vi "Station2_Data_Log_Bypass_Station1.vi"(8 "error in (no error)":errorcluster, 11 "Cluster 2":T2) -> (0 "error out":errorcluster)   [LabVIEW 2017]
uses:
  <vilib>/addons/database/Connection.llb/Conn ObjectReference.ctl
  <vilib>/addons/database/NI_Database_API.lvlib
panel:
  # "bypass station1 ..."
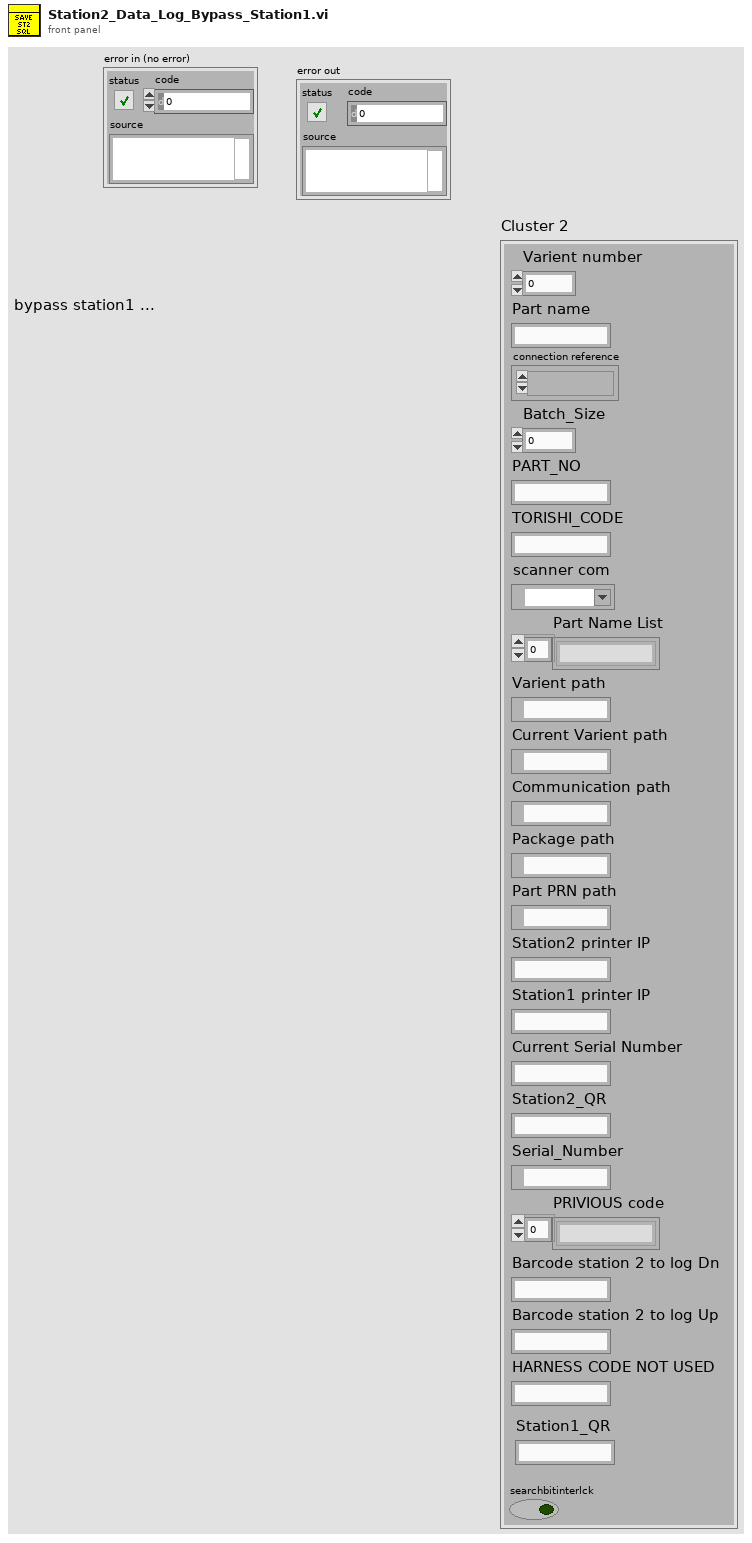
[diagram p1: front panel]
types:
  T1 = typedef "NI_Database_API.lvlib/Conn ObjectReference.ctl" = refnum<k1>
  T2 = cluster{"Varient number":u16, "Part name":string, "connection reference":T1, "Batch_Size":u16, "PART_NO":string, "TORISHI_CODE":string, "scanner com":refnum<visa-resource-name>, "Part Name List":string[], "Varient path":path, "Current Varient path":path, "Communication path":path, "Package path":path, "Part PRN path":path, "Station2 printer IP":string, "Station1 printer IP":string, "Current Serial Number":string, "Station2_QR":string, "Serial_Number":path, "PRIVIOUS code":string[], "Barcode station 2 to log Dn":string, "Barcode station 2 to log Up":string, "HARNESS CODE NOT USED":string, "Station1_QR":string, "searchbitinterlck":bool}
  T3 = cluster{"appended array[0]":string, "appended array[1]":string, "appended array[2]":string, "appended array[3]":string, "appended array[4]":string, "appended array[5]":string, "appended array[6]":string, "appended array[7]":string, "appended array[8]":string, "appended array[9]":string, "appended array[10]":string, "appended array[11]":string, "appended array[12]":string, "appended array[13]":string, "appended array[14]":string, "appended array[15]":string, "appended array[16]":string, "appended array[17]":string, "appended array[18]":string, "appended array[19]":string, "appended array[20]":string, "appended array[21]":string, "appended array[22]":string, "appended array[23]":string, "appended array[24]":string, "appended array[25]":string, "appended array[26]":string, "appended array[27]":string, "appended array[28]":string, "appended array[29]":string, "appended array[30]":string, "appended array[31]":string, "appended array[32]":string, "appended array[33]":string, "appended array[34]":string, "appended array[35]":string, "appended array[36]":string, "appended array[37]":string, "appended array[38]":string, "appended array[39]":string, "appended array[40]":string, "appended array[41]":string, "appended array[42]":string, "appended array[43]":string, "appended array[44]":string, "appended array[45]":string, "appended array[46]":string, "appended array[47]":string, "appended array[48]":string, "appended array[49]":string, "appended array[50]":string, "appended array[51]":string, "appended array[52]":string, "appended array[53]":string, "appended array[54]":string, "appended array[55]":string, "appended array[56]":string, "appended array[57]":string, "appended array[58]":string, "appended array[59]":string, "appended array[60]":string, "appended array[61]":string, "appended array[62]":string, "appended array[63]":string, "appended array[64]":string, "appended array[65]":string, "appended array[66]":string, "appended array[67]":string, "appended array[68]":string, "appended array[69]":string, "appended array[70]":string, "appended array[71]":string, "appended array[72]":string, "appended array[73]":string, "appended array[74]":string, "appended array[75]":string, "appended array[76]":string}
  T4 = typedef "LVDateTimeRec.ctl" = cluster{"fractional second":dbl, "second":i32, "minute":i32, "hour":i32, "day of month":i32, "month":i32, "year":i32, "day of week":i32, "day of year":i32, "DST":i32}
  T5 = cluster{"time stamp":timestamp, string, string, string, string, string, string, string, string, string, string, string, string, string, string, string, string, string, string, string, string, string, string, string, string, string, string, string, string, string, string, string, string, "time stamp":timestamp, "Station2_QR":string, string, string, "Numeric 2":string, "Numeric 2":string, "Numeric 2":string, string, "Numeric 2":string, "Numeric 2":string, string, "Numeric 2":string, "Numeric 2":string, "Numeric 2":string, string, "Numeric 2":string, "Numeric 2":string, "Numeric 2":string, string, "Numeric 2":string, "Numeric 2":string, "Numeric 2":string, string, "Numeric 2":string, "Numeric 2":string, "Numeric 2":string, string, "Numeric 2":string, "Numeric 2":string, "Numeric 2":string, string, "Numeric 2":string, "Numeric 2":string, "Numeric 2":string, string, string, string, string, string, string, string, string, string, string}
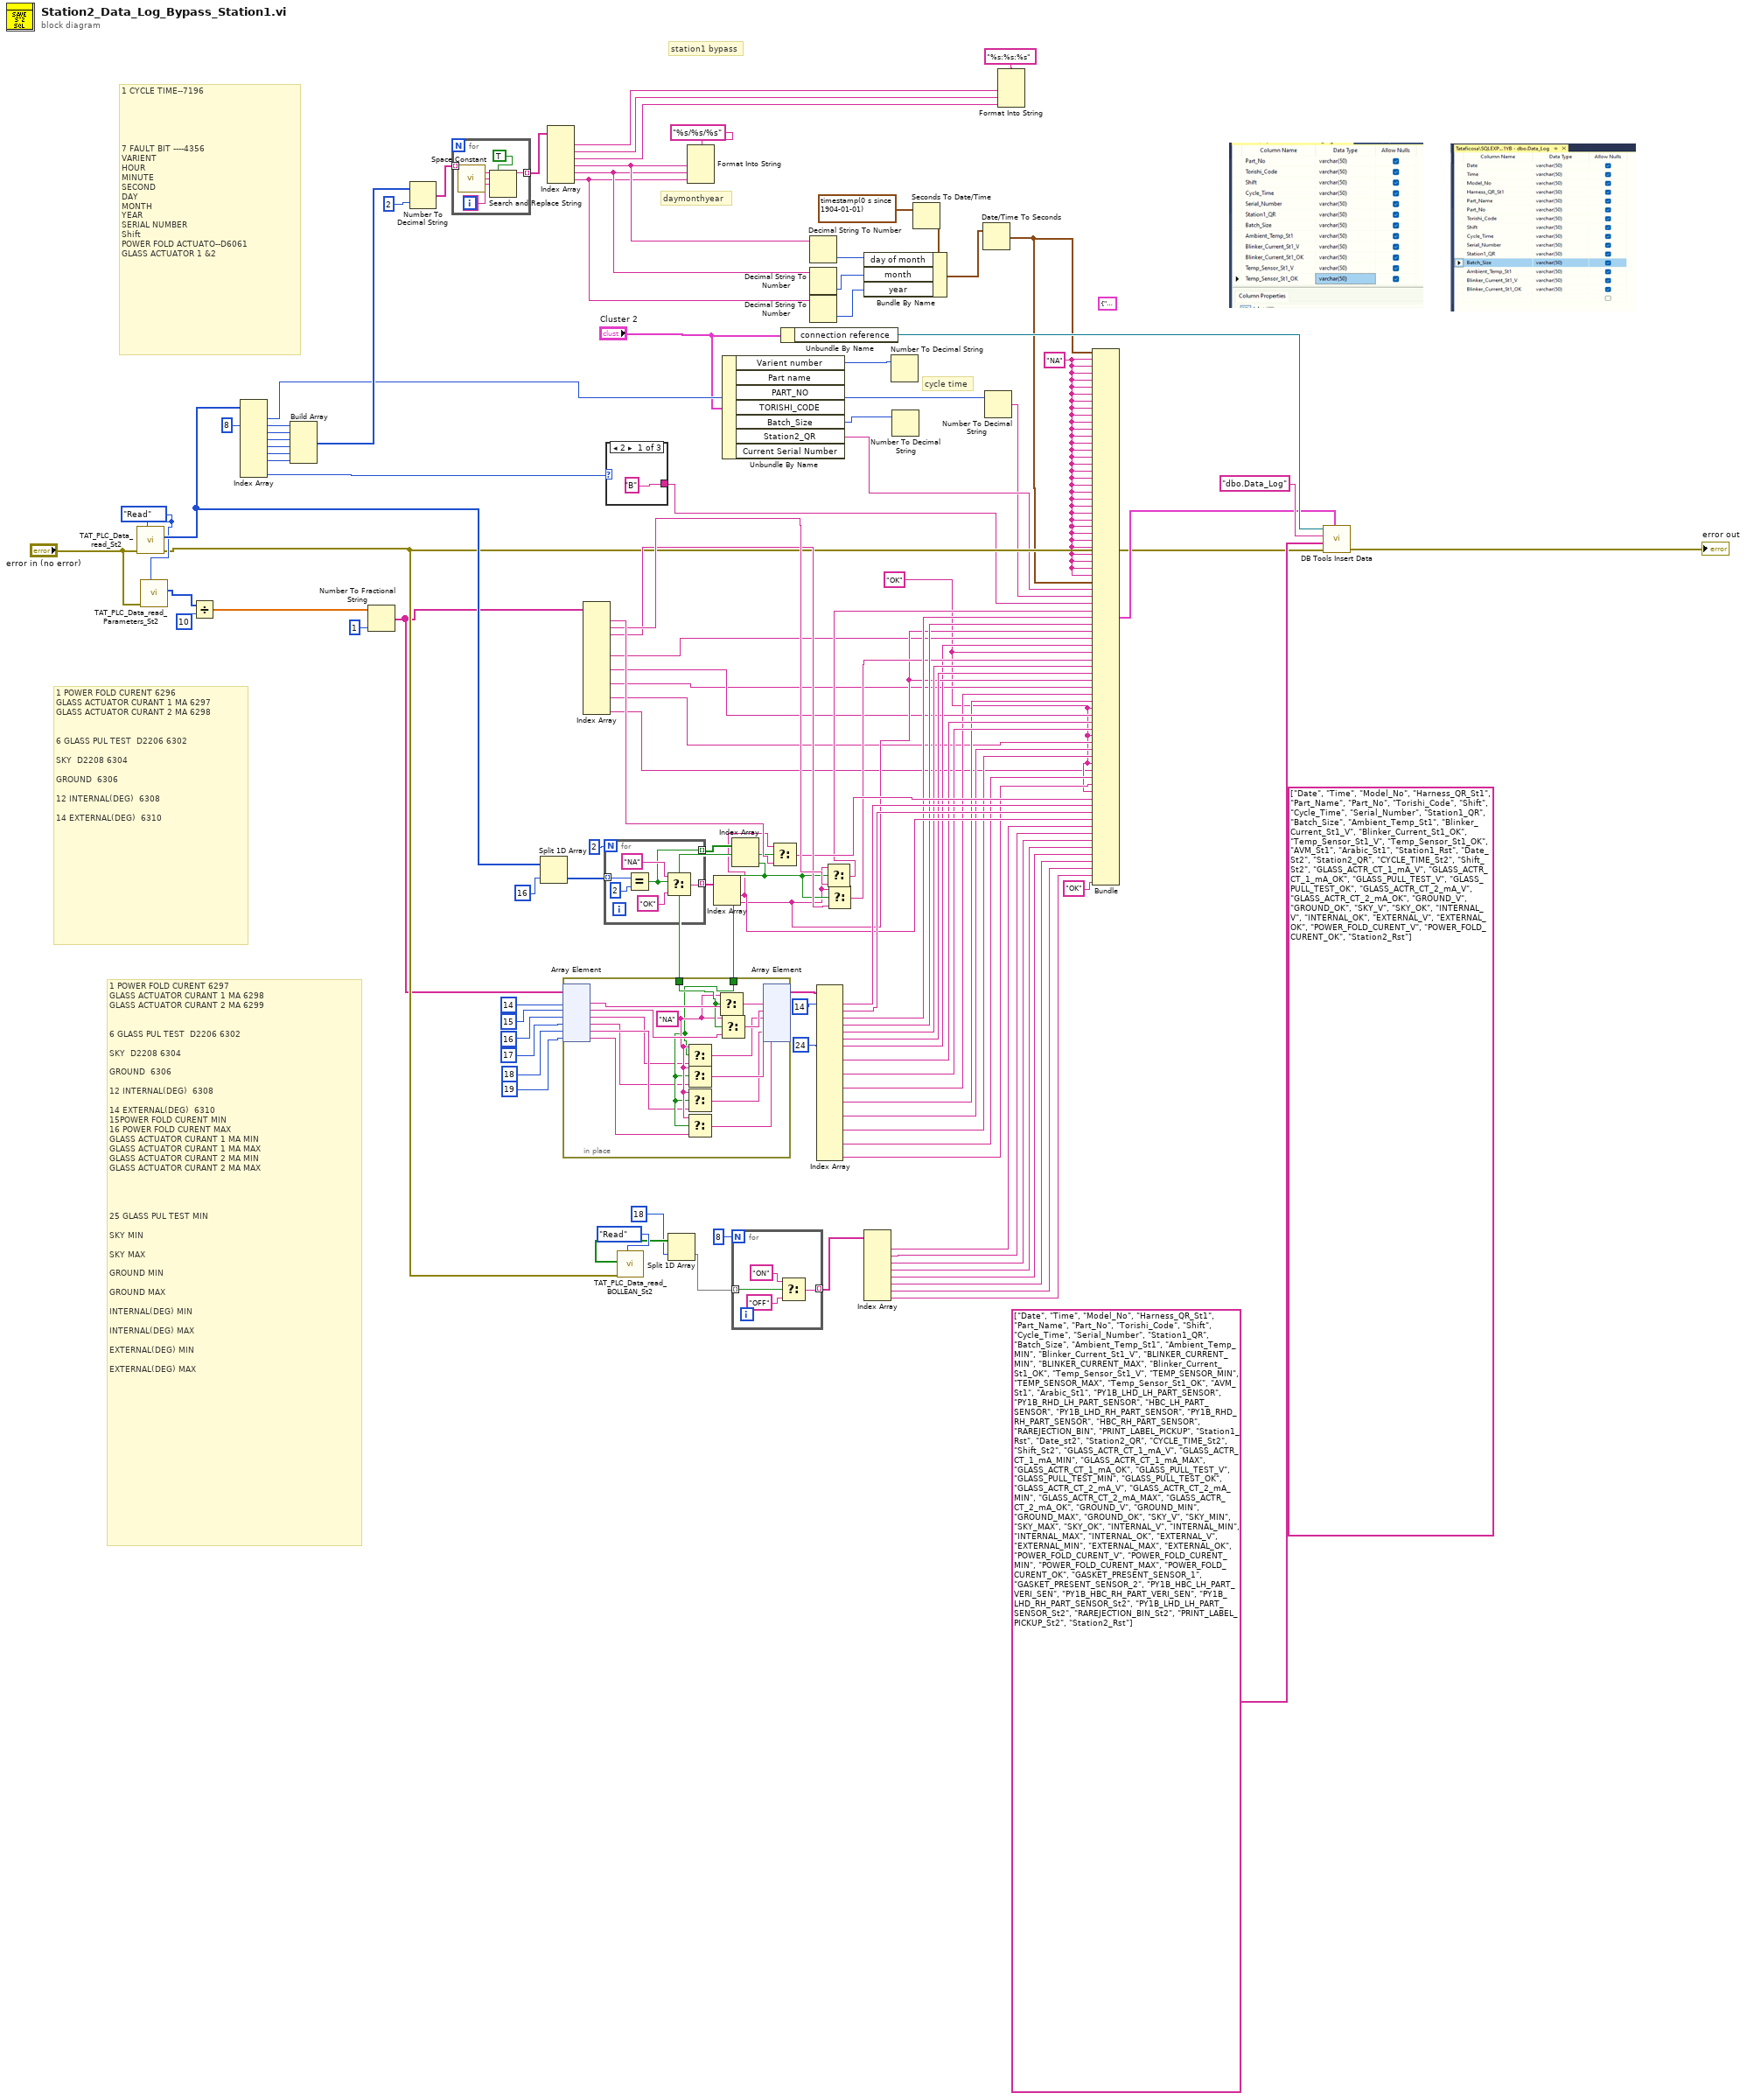
[diagram p0: block diagram]
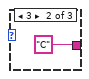
[diagram p2: hidden frame]
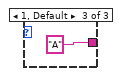
[diagram p3: hidden frame]
diagram:
  (unwired) T3 {"appended array[0]"="Date", "appended array[1]"="Time", "appended array[2]"="Model_No", "appended array[3]"="Harness_QR_St1", "appended array[4]"="Part_Name", "appended array[5]"="Part_No", "appended array[6]"="Torishi_Code", "appended array[7]"="Shift", "appended array[8]"="Cycle_Time", "appended array[9]"="Serial_Number", "appended array[10]"="Station1_QR", "appended array[11]"="Batch_Size", "appended array[12]"="Ambient_Temp_St1", "appended array[13]"="Ambient_Temp_MIN", "appended array[14]"="Blinker_Current_St1_V", "appended array[15]"="BLINKER_CURRENT_MIN", "appended array[16]"="BLINKER_CURRENT_MAX", "appended array[17]"="Blinker_Current_St1_OK", "appended array[18]"="Temp_Sensor_St1_V", "appended array[19]"="TEMP_SENSOR_MIN", "appended array[20]"="TEMP_SENSOR_MAX", "appended array[21]"="Temp_Sensor_St1_OK", "appended array[22]"="AVM_St1", "appended array[23]"="Arabic_St1", "appended array[24]"="PY1B_LHD_LH_PART_SENSOR", "appended array[25]"="PY1B_RHD_LH_PART_SENSOR", "appended array[26]"="HBC_LH_PART_SENSOR", "appended array[27]"="PY1B_LHD_RH_PART_SENSOR", "appended array[28]"="PY1B_RHD_RH_PART_SENSOR", "appended array[29]"="HBC_RH_PART_SENSOR", "appended array[30]"="RAREJECTION_BIN", "appended array[31]"="PRINT_LABEL_PICKUP", "appended array[32]"="Station1_Rst", "appended array[33]"="Date_st2", "appended array[34]"="Station2_QR", "appended array[35]"="CYCLE_TIME_St2", "appended array[36]"="Shift_St2", "appended array[37]"="GLASS_ACTR_CT_1_mA_V", "appended array[38]"="GLASS_ACTR_CT_1_mA_MIN", "appended array[39]"="GLASS_ACTR_CT_1_mA_MAX", "appended array[40]"="GLASS_ACTR_CT_1_mA_OK", "appended array[41]"="GLASS_PULL_TEST_V", "appended array[42]"="GLASS PUL TEST_MIN", "appended array[43]"="GLASS_PULL_TEST_OK", "appended array[44]"="GLASS_ACTR_CT_2_mA_V", "appended array[45]"="GLASS_ACTR_CT_2_mA_MIN", "appended array[46]"="GLASS_ACTR_CT_2_mA_MAX", "appended array[47]"="GLASS_ACTR_CT_2_mA_OK", "appended array[48]"="GROUND_V", "appended array[49]"="GROUND_MIN", "appended array[50]"="GROUND_MAX", "appended array[51]"="GROUND_OK", "appended array[52]"="SKY_V", "appended array[53]"="SKY_MIN", "appended array[54]"="SKY_MAX", "appended array[55]"="SKY_OK", "appended array[56]"="INTERNAL_V", "appended array[57]"="INTERNAL_MIN", "appended array[58]"="INTERNAL_MAX", "appended array[59]"="INTERNAL_OK", "appended array[60]"="EXTERNAL_V", "appended array[61]"="EXTERNAL_MIN", "appended array[62]"="EXTERNAL_MAX", "appended array[63]"="EXTERNAL_OK", "appended array[64]"="POWER_FOLD_CURENT_V", "appended array[65]"="POWER_FOLD_CURENT_MIN", "appended array[66]"="POWER_FOLD_CURENT_MAX", "appended array[67]"="POWER_FOLD_CURENT_OK", "appended array[68]"="GASKET_PRESENT_SENSOR_1", "appended array[69]"="GASKET_PRESENT_SENSOR_2", "appended array[70]"="PY1B_&_HBC_LH_PART_VERIFICATION_SENSOR_St2", "appended array[71]"="PY1B_&_HBC_RH_PART_VERIFICATION_SENSOR_St2", "appended array[72]"="PY1B_LHD_RH_PART_SENSOR_St2", "appended array[73]"="PY1B_LHD_LH_PART_SENSOR_St2", "appended array[74]"="RAREJECTION_BIN_St2", "appended array[75]"="PRINT_LABEL_PICKUP_St2", "appended array[76]"="Station2_Rst"} ("cluster")
  w2 = "NA"
  w16 = "OK"
  w78 = enum16{"Read", "Write"}."Read" ("Enum")
  (unwired) string[] ["Date", "Time", "Model_No", "Harness_QR_St1", "Part_Name", "Part_No", "Torishi_Code", "Shift", "Cycle_Time", "Serial_Number", "Station1_QR", "Batch_Size", "Ambient_Temp_St1", "Blinker_Current_St1_V", "Blinker_Current_St1_OK", "Temp_Sensor_St1_V", "Temp_Sensor_St1_OK", "AVM_St1", "Arabic_St1", "Station1_Rst", "Date_St2", "Station2_QR", "CYCLE_TIME_St2", "Shift_St2", "GLASS_ACTR_CT_1_mA_V", "GLASS_ACTR_CT_1_mA_OK", "GLASS_PULL_TEST_V", "GLASS_PULL_TEST_OK", "GLASS_ACTR_CT_2_mA_V", "GLASS_ACTR_CT_2_mA_OK", "GROUND_V", "GROUND_OK", "SKY_V", "SKY_OK", "INTERNAL_V", "INTERNAL_OK", "EXTERNAL_V", "EXTERNAL_OK", "POWER_FOLD_CURENT_V", "POWER_FOLD_CURENT_OK", "Station2_Rst"] ("columns")
  # "1 POWER FOLD CURENT 6297\nGLASS ACTUATOR CURANT 1 MA 6298\nGLASS ACTUATOR CURANT 2 MA 6299\n\n\n6 GLASS PUL TEST  D2206 6302\n\nSKY  D2208 6304\n\nGROUND  6306\n\n12 INTERNAL(DEG)  6308\n\n14 EXTERNAL(DEG)  6310\n15POWER FOLD CURENT MIN\n16 POWER FOLD CURENT MAX\nGLASS ACTUATOR CURANT 1 MA MIN\nGLASS ACTUATOR CURANT 1 MA MAX\nGLASS ACTUATOR CURANT 2 MA MIN\nGLASS ACTUATOR CURANT 2 MA MAX\n\n\n\n\n25 GLASS PUL TEST MIN\n\nSKY MIN\n\nSKY MAX\n\nGROUND MIN\n\nGROUND MAX\n\nINTERNAL(DEG) MIN\n\nINTERNAL(DEG) MAX\n\nEXTERNAL(DEG) MIN\n\nEXTERNAL(DEG) MAX"
  # "1 POWER FOLD CURENT 6296\nGLASS ACTUATOR CURANT 1 MA 6297\nGLASS ACTUATOR CURANT 2 MA 6298\n\n\n6 GLASS PUL TEST  D2206 6302\n\nSKY  D2208 6304\n\nGROUND  6306\n\n12 INTERNAL(DEG)  6308\n\n14 EXTERNAL(DEG)  6310"
  # "1 CYCLE TIME--7196\n\n\n\n\n\n7 FAULT BIT ----4356\nVARIENT\nHOUR\nMINUTE\nSECOND\nDAY\nMONTH\nYEAR\nSERIAL NUMBER\nShift\nPOWER FOLD ACTUATO--D6061\nGLASS ACTUATOR 1 &2"
  # "station1 bypass"
  # "daymonthyear"
  # "cycle time"
  n1 = call "TAT_PLC_Data_read_St2.vi"("Enum"=w78, "error in (no error)"="error in (no error)") -> ("error out"=w61:errorcluster, "Array 2"=w79:u16[])  [unwired: 8 in]
  n2 = call "TAT_PLC_Data_read_Parameters_St2.vi"("Enum"=w78, "error in (no error)"="error in (no error)") -> ("Array 2"=w76:u16[])  [unwired: 8 in, 1 out]
  n3 = Divide(x=w76, y=10 ("Numeric 2")) -> (x/y=w73:dbl[])
  n4 = Index Array(array=w79, index #2=8 ("index")) -> (element #1=w81:u16, element #2=w99:u16, element #3=w98:u16, element #4=w97:u16, element #5=w96:u16, element #6=w95:u16, element #7=w94:u16, element #9=w87:u16)  [unwired: 8 in, 1 out]
  n5 = Build Array(w99, w98, w97, w96, w95, w94) -> (w93:u16[])
  n6 = Number To Fractional String(number=w73, precision (6)=i16 1) -> (F-format string=w43:string[])  [unwired: 2 in]
  n7 = Number To Decimal String(number=w93, width (-)=i16 2) -> (decimal integer string=w102:string[])
  n8 = for {
    tunnel: w102 -> [w111] mode=indexing
    tunnel: [w110] -> w101 mode=indexing
    n9 = call <vilib>:"Space Constant.vi"() -> ("String"=w112:string)
    n10 = Search and Replace String(replace all?=TRUE ("replace all? (F)"), input string=w111, search string=w112, replace string="0" ("replace string (\"\")")) -> (result string=w110:string)  [unwired: 4 in, 3 out]
  }
  n11 = Split 1D Array(array=w79, index=16) -> (second subarray=w85:u16[])  [unwired: 1 out]
  n12 = Index Array(array=w101) -> (element #1=w91:string, element #2=w90:string, element #3=w89:string, element #4=w5:string, element #5=w4:string, element #6=w3:string)  [unwired: 6 in]
  n13 = Index Array(array=w43) -> (element #1=w72:string, element #2=w71:string, element #3=w70:string, element #6=w28:string, element #8=w25:string, element #10=w24:string, element #12=w21:string, element #14=w15:string)  [unwired: 14 in, 6 out]
  n14 = for {
    N: 2 -> [_]
    tunnel: w85 -> [w120] mode=indexing
    tunnel: [w116] -> w83 mode=indexing
    tunnel: [w115] -> w82 mode=indexing
    n15 = Equal?(x=w120, y=2) -> (x = y?=w115:bool)
    n16 = Select(t="NA", s=w115, f="OK") -> (s? t:f=w116:string)
  }
  n17 = case shown="2" w87 {
    tunnel: ["B" "C" "A"] -> w12
    frame 2 {
    }
    frame 3 {
    }
    frame 1, Default {
    }
  }
  n18 = call "TAT_PLC_Data_read_BOLLEAN_St2.vi"("Enum"=enum16{"Read", "Write"}."Read", "error in (no error)"=w61) -> ("Array 2"=w66:bool[])  [unwired: 8 in, 1 out]
  n19 = Split 1D Array(array=w66, index=18) -> (second subarray=w64:bool[])  [unwired: 1 out]
  n20 = Format Into String(format string="%s/%s/%s" ("time format string (%c)"), w5, w4, w3) -> ()  [unwired: 2 in, 2 out]
  n21 = Index Array(array=w83) -> (element #1=w38:string, element #2=w30:string)  [unwired: 2 in]
  n22 = Unbundle By Name("Cluster 2") -> ("Varient number"=w108:u16, "Batch_Size"=w109:u16, "Station2_QR"=w14:string)  [unwired: 4 out]
  n23 = Index Array(array=w82) -> (element #1=w42:bool, element #2=w41:bool)  [unwired: 2 in]
  n24 = in-place {
    in-place-border: w41 -> [w132]
    in-place-border: w42 -> [w134]
    w133 = "NA"
    n25 = in-place-array #1(w43, 14 ("index"), 15 ("index"), 16 ("index"), 17 ("index"), 18 ("index"), 19 ("index")) -> (w138:string, w135:string, w128:string, w129:string, w130:string, w131:string)
    n26 = Select(t=w133, s=w132, f=w128) -> (s? t:f=w127:string)
    n27 = Select(t=w133, s=w132, f=w129) -> (s? t:f=w126:string)
    n28 = Select(t=w133, s=w132, f=w130) -> (s? t:f=w125:string)
    n29 = Select(t=w133, s=w132, f=w131) -> (s? t:f=w124:string)
    n30 = Select(t=w133, s=w134, f=w138) -> (s? t:f=w137:string)
    n31 = Select(t=w133, s=w134, f=w135) -> (s? t:f=w136:string)
    n32 = in-place-array #1(w137, w136, w127, w126, w125, w124) -> (w45:string[])  [unwired: 6 out]
  }
  n33 = for {
    N: 8 -> [_]
    tunnel: w64 -> [w140] mode=indexing
    tunnel: [w139] -> w62 mode=indexing
    n34 = Select(t="ON", s=w140, f="OFF") -> (s? t:f=w139:string)
  }
  n35 = Select(t=w38, s=w42, f=w72) -> (s? t:f=w37:string)
  n36 = Unbundle By Name("Cluster 2") -> ("connection reference"=w107:T1)
  n37 = Decimal String To Number(string=w5) -> (number=w9:i32)  [unwired: 2 in, 1 out]
  n38 = Decimal String To Number(string=w4) -> (number=w8:i32)  [unwired: 2 in, 1 out]
  n39 = Decimal String To Number(string=w3) -> (number=w7:i32)  [unwired: 2 in, 1 out]
  n40 = Index Array(array=w45, index #1=14 ("index"), index #7=24 ("index")) -> (element #1=w40:string, element #2=w39:string, element #3=w36:string, element #4=w35:string, element #5=w33:string, element #6=w32:string, element #7=w29:string, element #9=w27:string, element #11=w26:string, element #13=w23:string, element #15=w22:string, element #17=w20:string, element #19=w19:string, element #21=w18:string, element #23=w17:string)  [unwired: 21 in, 8 out]
  n41 = Select(t=w30, s=w41, f=w71) -> (s? t:f=w34:string)
  n42 = Select(t=w30, s=w41, f=w70) -> (s? t:f=w31:string)
  n43 = Index Array(array=w62) -> (element #1=w53:string, element #2=w54:string, element #3=w55:string, element #4=w56:string, element #5=w57:string, element #6=w58:string, element #7=w59:string, element #8=w60:string)  [unwired: 8 in]
  n44 = Number To Decimal String(number=w108) -> ()  [unwired: 1 in, 1 out]
  n45 = Number To Decimal String(number=w109) -> ()  [unwired: 1 in, 1 out]
  n46 = Seconds To Date/Time(time stamp (now)=timestamp(0 s since 1904-01-01)) -> (date time rec=w11:T4)  [unwired: 1 in]
  n47 = Bundle By Name(cluster=w11, "day of month"=w9, "month"=w8, "year"=w7) -> (w10:T4)
  n48 = Date/Time To Seconds(2:w10) -> (0:w1:timestamp)  [unwired: 1 in]
  n49 = Number To Decimal String(number=w81) -> (decimal integer string=w13:string)  [unwired: 1 in]
  n50 = Format Into String(format string="%s:%s:%s" ("time format string (%c)"), w91, w90, w89) -> ()  [unwired: 2 in, 2 out]
  n51 = Bundle("time stamp"=w1, w2, w2, w2, w2, w2, w2, w2, w2, w2, w2, w2, w2, w2, w2, w2, w2, w2, w2, w2, w2, w2, w2, w2, w2, w2, w2, w2, w2, w2, w2, w2, w2, "time stamp"=w1, "Station2_QR"=w14, w13, w12, "Numeric 2"=w34, "Numeric 2"=w36, "Numeric 2"=w35, w30, "Numeric 2"=w28, "Numeric 2"=w29, w16, "Numeric 2"=w31, "Numeric 2"=w33, "Numeric 2"=w32, w30, "Numeric 2"=w24, "Numeric 2"=w23, "Numeric 2"=w22, w16, "Numeric 2"=w25, "Numeric 2"=w27, "Numeric 2"=w26, w16, "Numeric 2"=w21, "Numeric 2"=w20, "Numeric 2"=w19, w16, "Numeric 2"=w15, "Numeric 2"=w18, "Numeric 2"=w17, w16, "Numeric 2"=w37, "Numeric 2"=w40, "Numeric 2"=w39, w38, w53, w54, w55, w56, w57, w58, w59, w60, "OK") -> (w104:T5)  [unwired: 1 in]
  n52 = call <vilib>:"DB Tools Insert Data.vi"("data"=w104, "error in (no error)"=w61, "columns"=string[] ["Date", "Time", "Model_No", "Harness_QR_St1", "Part_Name", "Part_No", "Torishi_Code", "Shift", "Cycle_Time", "Serial_Number", "Station1_QR", "Batch_Size", "Ambient_Temp_St1", "Ambient_Temp_MIN", "Blinker_Current_St1_V", "BLINKER_CURRENT_MIN", "BLINKER_CURRENT_MAX", "Blinker_Current_St1_OK", "Temp_Sensor_St1_V", "TEMP_SENSOR_MIN", "TEMP_SENSOR_MAX", "Temp_Sensor_St1_OK", "AVM_St1", "Arabic_St1", "PY1B_LHD_LH_PART_SENSOR", "PY1B_RHD_LH_PART_SENSOR", "HBC_LH_PART_SENSOR", "PY1B_LHD_RH_PART_SENSOR", "PY1B_RHD_RH_PART_SENSOR", "HBC_RH_PART_SENSOR", "RAREJECTION_BIN", "PRINT_LABEL_PICKUP", "Station1_Rst", "Date_st2", "Station2_QR", "CYCLE_TIME_St2", "Shift_St2", "GLASS_ACTR_CT_1_mA_V", "GLASS_ACTR_CT_1_mA_MIN", "GLASS_ACTR_CT_1_mA_MAX", "GLASS_ACTR_CT_1_mA_OK", "GLASS_PULL_TEST_V", "GLASS_PULL_TEST_MIN", "GLASS_PULL_TEST_OK", "GLASS_ACTR_CT_2_mA_V", "GLASS_ACTR_CT_2_mA_MIN", "GLASS_ACTR_CT_2_mA_MAX", "GLASS_ACTR_CT_2_mA_OK", "GROUND_V", "GROUND_MIN", "GROUND_MAX", "GROUND_OK", "SKY_V", "SKY_MIN", "SKY_MAX", "SKY_OK", "INTERNAL_V", "INTERNAL_MIN", "INTERNAL_MAX", "INTERNAL_OK", "EXTERNAL_V", "EXTERNAL_MIN", "EXTERNAL_MAX", "EXTERNAL_OK", "POWER_FOLD_CURENT_V", "POWER_FOLD_CURENT_MIN", "POWER_FOLD_CURENT_MAX", "POWER_FOLD_CURENT_OK", "GASKET_PRESENT_SENSOR_1", "GASKET_PRESENT_SENSOR_2", "PY1B_HBC_LH_PART_VERI_SEN", "PY1B_HBC_RH_PART_VERI_SEN", "PY1B_LHD_RH_PART_SENSOR_St2", "PY1B_LHD_LH_PART_SENSOR_St2", "RAREJECTION_BIN_St2", "PRINT_LABEL_PICKUP_St2", "Station2_Rst"] ("appended array"), "table"="dbo.Data_Log", "connection reference"=w107) -> ("error out"=→"error out":errorcluster)  [unwired: 5 in, 1 out]
